vi "GetImageSize.vi"(0 "reference in":refnum<class "LcPictureBox.lvclass">, 5 "error in (no error)":errorcluster) -> (14 "reference out":refnum<class "LcPictureBox.lvclass">, 16 "Width":i32, 17 "Height":i32, 19 "error out":errorcluster)   [LabVIEW 2020, in "LcPictureBox.lvclass"]
uses:
  LcPictureBox.lvclass
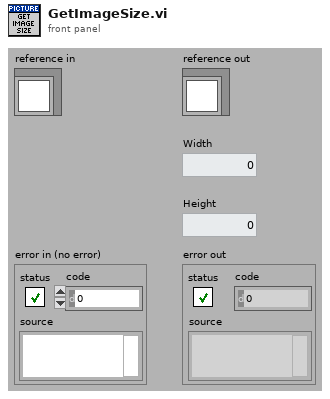
[diagram p1: front panel]
types:
  T1 = typedef "LcPictureBox.lvclass/ObjectAttributes.ctl" = cluster{"PictureBox":refnum<k24>, "ImageSize":cluster{"Width":i32, "Height":i32}, "PenMemory":map{cluster{"Alpha(100%)":dbl, "Color(Black)":u32, "Pen(Width=1, Solid)":T2}, refnum<k24>}, "GraphicsRef":refnum<k24>, "BrushMemory":map{cluster{"Alpha(100%)":dbl, "Color(Black)":u32}, refnum<k24>}, "Images":refnum<k24>[], "ImageIndex":i32, "BgColor(None)":u32, "LoadedImages":map{string, cluster{"ImageOut":refnum<k24>, "ImageSize":cluster{"Width":i32, "Height":i32}}}, "ColorsMemory":map{cluster{"Alpha(100%)":dbl, "Color(Black)":u32}, refnum<k24>}, "CacheSize":i32, "PictureBoxActiveXReference":refnum<vi>, "Scale":sgl, "Offset":cluster{"x":sgl, "y":sgl}, "zoom_center":cluster{"X":i32, "Y":i32}, "ImagesCreated":refnum<k24>[]}
  T2 = typedef "LcPictureBox.lvclass/Pen.ctl" = cluster{"Width":u16, "Style":enum32{"Solid", "Dash", "Dot", "DashDot", "DashDotDot"}}
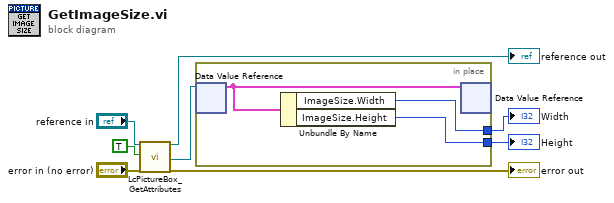
[diagram p0: block diagram]
diagram:
  n1 = call "LcPictureBox_GetAttributes.vi"("reference in"="reference in", "OnlyGetDvrReference(False)"=TRUE, "error in (no error)"="error in (no error)") -> ("reference out"=→"reference out":refnum<class "LcPictureBox.lvclass">, "DataRef"=w2:refnum<data-value>, "error out"=→"error out":errorcluster)  [unwired: 13 in, 1 out]
  n2 = in-place {
    in-place-border: [w11] -> w4
    in-place-border: [w9] -> w1
    n3 = in-place-dvr #1(w2) -> (w10:T1)  [unwired: 1 out]
    n4 = Unbundle By Name(w10) -> ("ImageSize.Width"=w11:i32, "ImageSize.Height"=w9:i32)
    n5 = in-place-dvr #1(w10) -> ()  [unwired: 2 out]
  }
  "Width" <- w4
  "Height" <- w1
